vi "Module Init.vi"(8 "error in (no error)":errorcluster, 11 "GenericGuiAO in":refnum<class "GenericGuiDO.lvclass">) -> (0 "error out":errorcluster, 3 "GenericGuiAO out":refnum<class "GenericGuiDO.lvclass">)   [LabVIEW 2020, in "VolatusDAQGenericGUI.lvlib" / "GenericGuiDO.lvclass"]
uses:
  GenericGuiDO.lvclass
  C:/dev/lv20CE/relink/lv-volatus/Volatus/Module/Module.lvclass
  VolatusConfig/Meta Type.ctl
  VolatusConfig/Meta Name.ctl
  Volatus/Module/Module.lvclass/Module.ctl
  VolatusConfig/VolatusConfigElement/VolatusConfigElement.lvclass/VolatusConfigElement.ctl
  GenericGuiDO.lvclass/GenericGuiDO.ctl
  VolatusConfig/VolatusConfigElement/Element.vi
  lv-cdm/CDM-Config/Config Lookup/Match Meta.vi
  lv-cdm/CDM-Config/Config Element/Owner.vi
  lv-cdm/CDM-Config/Config Manager/Lookup Descendant.vi
  VolatusConfig/Group/Group.lvclass
  lv-cdm/CDM-Config/Config Filter/Config Lookup.lvclass
  Volatus/Module/Module.lvclass
  VolatusConfig/VolatusConfigElement/VolatusConfigElement.lvclass
  VolatusConfig/VolatusConfig.lvlib
  lv-cdm/CDM-Config/Config Element/Config Element.lvclass
  VolatusConfig/Task/Task.lvclass
  C:/dev/lv20CE/relink/lv-volatus/VolatusDAQGenericGUI/GenericGuiDO/GenericGuiDO.lvclass
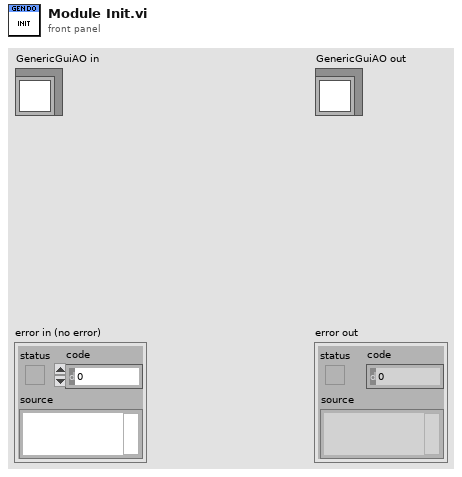
[diagram p1: front panel]
types:
  T1 = typedef "VolatusConfig.lvlib/Meta Name.ctl" = enum16{"VL_Type", "VL_Node_IP", "VL_Node_Type", "VL_Task_Type", "VL_Group_Type", "VL_Channel_Type", "VL_Channel_DataType", "VL_Config_Version", "VL_Overlay_Type"}
  T2 = typedef "VolatusConfig.lvlib/Meta Type.ctl" = enum16{"UNKNOWN", "VL_System", "VL_Cluster", "VL_Node", "VL_Task", "VL_Group", "VL_Channel", "VL_Task_List", "VL_Scaling", "VL_Sensor", "VL_Sensor_List", "VL_Scale"}
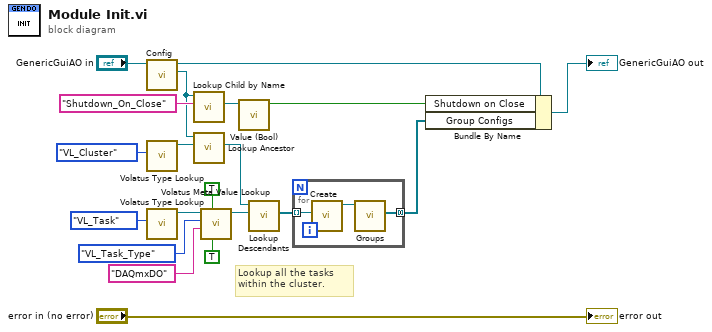
[diagram p0: block diagram]
diagram:
  # "Lookup all the tasks within the cluster."
  n1 = call "Config.vi"("Module in"="GenericGuiAO in") -> ("Config"=w2:refnum<class "VolatusConfigElement.lvclass">, "Module out"=w7:refnum<class "GenericGuiDO.lvclass">)  [unwired: 9 in]
  n2 = call "Volatus Type Lookup.vi"("Meta Type"=Meta_Type."VL_Cluster") -> ("Config Lookup out"=w19:refnum<class "Config Lookup.lvclass">)  [unwired: 9 in, 1 out]
  n3 = call "Volatus Type Lookup.vi"("Meta Type"=Meta_Type."VL_Task") -> ("Config Lookup out"=w15:refnum<class "Config Lookup.lvclass">)  [unwired: 9 in, 1 out]
  n4 = call "Lookup Child by Name.vi"("Child Name"="Shutdown_On_Close", "VolatusConfigElement in"=w2) -> ("Child"=w3:refnum<class "Config Element.lvclass">)  [unwired: 6 in, 3 out]
  n5 = call "Lookup Ancestor.vi"("Lookup"=w19, "VolatusConfigElement in"=w2) -> ("Ancestor"=w17:refnum<class "Config Element.lvclass">)  [unwired: 7 in, 2 out]
  n6 = call "Volatus Meta Value Lookup.vi"("Exact Value (F)"=TRUE, "Don't Recurse Past Match (F)"=TRUE, "Value"="DAQmxDO", "Meta Name"=Meta_Name."VL_Task_Type", "Config Lookup (New)"=w15) -> ("Config Lookup out"=w11:refnum<class "Config Lookup.lvclass">)  [unwired: 5 in, 1 out]
  n7 = call "Value (Bool).vi"("Config Element in"=w3) -> ("Bool Value"=w1:bool)  [unwired: 9 in, 1 out]
  n8 = call "Lookup Descendants.vi"("Lookup"=w11, "Config Element in"=w17) -> ("Descendants"=w10:refnum<class "Config Element.lvclass">[])  [unwired: 7 in, 2 out]
  n9 = for {
    tunnel: w10 -> [w23] mode=indexing
    tunnel: [w21] -> w5 mode=concatenating
    n10 = call "Create.vi"("Element"=w23) -> ("Task out"=w22:refnum<class "Task.lvclass">)  [unwired: 9 in, 1 out]
    n11 = call "Groups.vi"("Task in"=w22) -> ("Groups"=w21:refnum<class "Group.lvclass">[])  [unwired: 8 in, 2 out]
  }
  n12 = Bundle By Name(cluster=w7, "Shutdown on Close"=w1, "Group Configs"=w5) -> (→"GenericGuiAO out":refnum<class "GenericGuiDO.lvclass">)
  "error out" <- "error in (no error)"
